vi "StartUp Sequence Open Loop Rev 1.1.vi"() -> ()   [LabVIEW 2017]
panel:
  in  "Shut Off":bool
  out "ECU COM Port Out":refnum<visa-resource-name>
  out "Throttle Position":string
  out "Turbine RPM":string
  out "Turbine Temp":string
  out "Pump Voltage":string
  out "Error Out":errorcluster
  in  "Error In":errorcluster
  in  "ECU COM Port":refnum<visa-resource-name>
  out "Turbine State":string
  in  "Strt Sqnc":bool
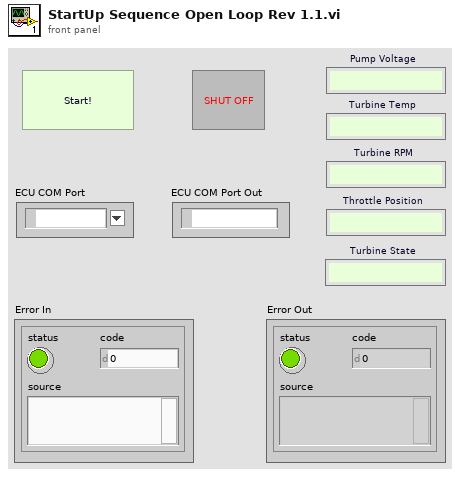
[diagram p1: front panel]
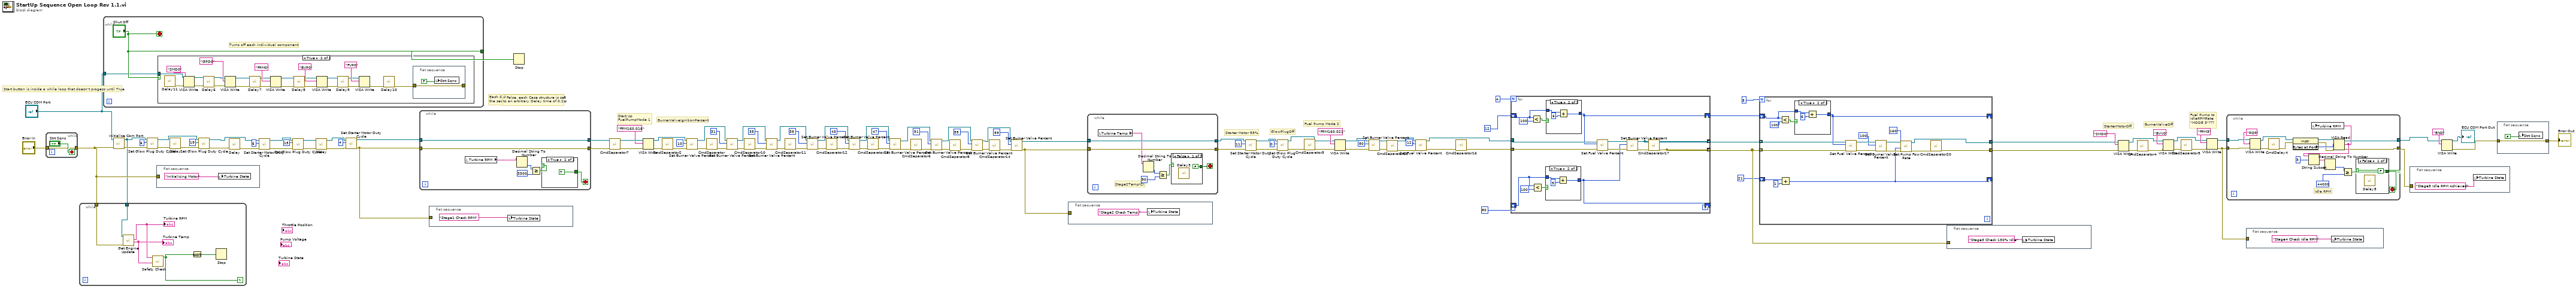
[diagram p0: block diagram]
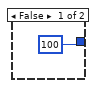
[diagram p2: hidden frame]
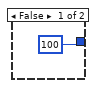
[diagram p3: hidden frame]
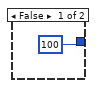
[diagram p4: hidden frame]
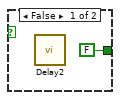
[diagram p6: hidden frame]
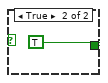
[diagram p7: hidden frame]
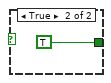
[diagram p8: hidden frame]
diagram:
  # "Start button is inside a while loop that doesn't progess until True"
  # "Fuel Pump Mode 2"
  # "Starter Motor 55%"
  # "Fuel Pump to \nIdleRPMRate\n\"MODE 3\"???"
  # "BurnerValveOff"
  # "StarterMotorOff"
  # "GlowPlugOff"
  # "Start Up\nFuelPumpMode 1"
  # "BurnerValveIgnitionPercent"
  # "If False, each Case structure is set\nto an arbitrary Delay time of 0.2 s"
  # "Each Stage is inside a while loop so that \nthe sequence doesn't progress until True"
  n1 = while {
    tunnel: "Error In" -> [w114]
    tunnel: [w114] -> w2
    stop <- "Strt Sqnc" stop-if-true
  }
  n2 = while {
    tunnel: ["Shut Off"] -> w90
    tunnel: "ECU COM Port" -> [w116]
    stop <- "Shut Off" stop-if-true
    # "Turns off each individual component"
    n3 = case shown="True" "Shut Off" {
      tunnel: w116 -> [_ w120]
      frame False {
      }
      frame True {
        n4 = call "Delay11"() -> ("error out"=w118:errorcluster)  [unwired: 11 in]
        n5 = VISA Write(VISA resource name=w120, write buffer="SMD0", error in (no error)=w118) -> (VISA resource name out=w125:refnum<visa-resource-name>, error out=w138:errorcluster)  [unwired: 1 out]
        n6 = call "Delay6"("error in (no error)"=w138) -> ("error out"=w132:errorcluster)  [unwired: 10 in]
        n7 = VISA Write(VISA resource name=w125, write buffer="GPD0", error in (no error)=w132) -> (VISA resource name out=w123:refnum<visa-resource-name>, error out=w136:errorcluster)  [unwired: 1 out]
        n8 = call "Delay7"("error in (no error)"=w136) -> ("error out"=w131:errorcluster)  [unwired: 10 in]
        n9 = VISA Write(VISA resource name=w123, write buffer="FPM0", error in (no error)=w131) -> (VISA resource name out=w122:refnum<visa-resource-name>, error out=w135:errorcluster)  [unwired: 1 out]
        n10 = call "Delay8"("error in (no error)"=w135) -> ("error out"=w130:errorcluster)  [unwired: 10 in]
        n11 = VISA Write(VISA resource name=w122, write buffer="BVP0", error in (no error)=w130) -> (VISA resource name out=w121:refnum<visa-resource-name>, error out=w134:errorcluster)  [unwired: 1 out]
        n12 = call "Delay9"("error in (no error)"=w134) -> ("error out"=w129:errorcluster)  [unwired: 10 in]
        n13 = VISA Write(VISA resource name=w121, write buffer="FVP0", error in (no error)=w129) -> (error out=w133:errorcluster)  [unwired: 2 out]
        n14 = call "Delay10"("error in (no error)"=w133) -> ("error out"=w119:errorcluster)  [unwired: 10 in]
        n15 = flat-sequence {
          tunnel: w119 -> [w139]
          tunnel: [w139] -> _
          frame #0 {
            n16 = local write "Strt Sqnc"(FALSE ("Strt Sqnc")) -> ()
          }
        }
      }
    }
  }
  n17 = call "Initialize Com Port.vi"("Error In"=w2, "ECU COM Port"="ECU COM Port") -> ("Error Out"=w80:errorcluster, "ECU COM Port Out"=w1:refnum<visa-resource-name>)  [unwired: 8 in]
  n18 = while {
    tunnel: w2 -> [w146]
    tunnel: w1 -> [w145]
    stop <- w142 continue-if-true
    n19 = call "Get Engine Update.vi"("Error In"=w146, "ECU COM Port"=w145) -> ("Temperature"=w143:string, "RPMs"=w144:string)  [unwired: 6 in, 2 out]
    "Turbine RPM" <- w144
    "Turbine Temp" <- w143
    n20 = call "Safety Check.vi"("Temperature"=w143, "RPMs"=w144) -> ("Safe?"=w142:bool)  [unwired: 9 in]
    n21 = Not(x=w142) -> (.not. x?=w141:bool)
    n22 = Stop(stop? (T)=w141) -> ()
  }
  n23 = call "Set Glow Plug Duty Cycle.vi"("Error In"=w80, "Duty Cycle"=6, "ECU COM Port"=w1) -> ("Error Out"=w79:errorcluster, "ECU COM Port Out"=w76:refnum<visa-resource-name>)  [unwired: 7 in]
  n24 = flat-sequence {
    tunnel: w2 -> [_]
    frame #0 {
      n25 = local write "Turbine State"("Initializing Motor") -> ()
    }
  }
  n26 = call "Delay"("error in (no error)"=w79) -> ("error out"=w78:errorcluster)  [unwired: 10 in]
  n27 = call "Set Glow Plug Duty Cycle.vi"("Error In"=w78, "Duty Cycle"=19, "ECU COM Port"=w76) -> ("Error Out"=w77:errorcluster, "ECU COM Port Out"=w72:refnum<visa-resource-name>)  [unwired: 7 in]
  n28 = call "Delay"("error in (no error)"=w77) -> ("error out"=w73:errorcluster)  [unwired: 10 in]
  n29 = call "Set Starter Motor Duty Cycle.vi"("Error In"=w73, "Duty Cycle"=6, "ECU COM Port"=w72) -> ("Error Out"=w71:errorcluster, "ECU COM Port Out"=w69:refnum<visa-resource-name>)  [unwired: 7 in]
  n30 = call "Set Glow Plug Duty Cycle.vi"("Error In"=w71, "Duty Cycle"=15, "ECU COM Port"=w69) -> ("Error Out"=w70:errorcluster, "ECU COM Port Out"=w66:refnum<visa-resource-name>)  [unwired: 7 in]
  n31 = call "Delay"("error in (no error)"=w70) -> ("error out"=w67:errorcluster)  [unwired: 10 in]
  n32 = call "Set Starter Motor Duty Cycle.vi"("Error In"=w67, "Duty Cycle"=4, "ECU COM Port"=w66) -> ("Error Out"=w91:errorcluster, "ECU COM Port Out"=w65:refnum<visa-resource-name>)  [unwired: 7 in]
  n33 = while {
    tunnel: w91 -> [w150]
    tunnel: w65 -> [w149]
    tunnel: [w149] -> w101
    tunnel: [w150] -> w100
    stop <- w153 stop-if-true
    n34 = local read "Turbine RPM"() -> (w148:string)
    n35 = Decimal String To Number(string=w148) -> (number=w152:i32)  [unwired: 2 in, 1 out]
    n36 = Greater Or Equal?(x=w152, y=3300) -> (x >= y?=w154:bool)
    n37 = case shown="True" w154 {
      tunnel: [FALSE TRUE] -> w153
      frame False {
        n38 = call "Delay2"() -> ()  [unwired: 11 in, 1 out]
      }
      frame True {
      }
    }
  }
  n39 = flat-sequence {
    tunnel: w91 -> [_]
    frame #0 {
      n40 = local write "Turbine State"("Stage1 Check RPM") -> ()
    }
  }
  n41 = Stop(stop? (T)=w90) -> ()
  n42 = call "CmdSeparator7"("error in (no error)"=w100) -> ("error out"=w99:errorcluster)  [unwired: 10 in]
  n43 = VISA Write(VISA resource name=w101, write buffer="FPM160,016", error in (no error)=w99) -> (VISA resource name out=w53:refnum<visa-resource-name>, error out=w112:errorcluster)  [unwired: 1 out]
  n44 = call "CmdSeparator2"("error in (no error)"=w112) -> ("error out"=w64:errorcluster)  [unwired: 10 in]
  n45 = call "Set Burner Valve Percent.vi"("Error In"=w64, "Percent"=10, "ECU COM Port"=w53) -> ("Error Out"=w63:errorcluster, "ECU COM Port Out"=w52:refnum<visa-resource-name>)  [unwired: 7 in]
  n46 = call "CmdSeparator"("error in (no error)"=w63) -> ("error out"=w62:errorcluster)  [unwired: 10 in]
  n47 = call "Set Burner Valve Percent.vi"("Error In"=w62, "Percent"=31, "ECU COM Port"=w52) -> ("Error Out"=w61:errorcluster, "ECU COM Port Out"=w51:refnum<visa-resource-name>)  [unwired: 7 in]
  n48 = call "CmdSeparator10"("error in (no error)"=w61) -> ("error out"=w60:errorcluster)  [unwired: 10 in]
  n49 = call "Set Burner Valve Percent.vi"("Error In"=w60, "Percent"=35, "ECU COM Port"=w51) -> ("Error Out"=w59:errorcluster, "ECU COM Port Out"=w50:refnum<visa-resource-name>)  [unwired: 7 in]
  n50 = call "CmdSeparator11"("error in (no error)"=w59) -> ("error out"=w58:errorcluster)  [unwired: 10 in]
  n51 = call "Set Burner Valve Percent.vi"("Error In"=w58, "Percent"=39, "ECU COM Port"=w50) -> ("Error Out"=w57:errorcluster, "ECU COM Port Out"=w49:refnum<visa-resource-name>)  [unwired: 7 in]
  n52 = call "CmdSeparator12"("error in (no error)"=w57) -> ("error out"=w56:errorcluster)  [unwired: 10 in]
  n53 = call "Set Burner Valve Percent.vi"("Error In"=w56, "Percent"=43, "ECU COM Port"=w49) -> ("Error Out"=w55:errorcluster, "ECU COM Port Out"=w48:refnum<visa-resource-name>)  [unwired: 7 in]
  n54 = call "CmdSeparator13"("error in (no error)"=w55) -> ("error out"=w54:errorcluster)  [unwired: 10 in]
  n55 = call "Set Burner Valve Percent.vi"("Error In"=w54, "Percent"=47, "ECU COM Port"=w48) -> ("Error Out"=w24:errorcluster, "ECU COM Port Out"=w23:refnum<visa-resource-name>)  [unwired: 7 in]
  n56 = call "CmdSeparator6"("error in (no error)"=w24) -> ("error out"=w26:errorcluster)  [unwired: 10 in]
  n57 = call "Set Burner Valve Percent.vi"("Error In"=w26, "Percent"=51, "ECU COM Port"=w23) -> ("Error Out"=w19:errorcluster, "ECU COM Port Out"=w20:refnum<visa-resource-name>)  [unwired: 7 in]
  n58 = call "CmdSeparator8"("error in (no error)"=w19) -> ("error out"=w22:errorcluster)  [unwired: 10 in]
  n59 = call "Set Burner Valve Percent.vi"("Error In"=w22, "Percent"=55, "ECU COM Port"=w20) -> ("Error Out"=w15:errorcluster, "ECU COM Port Out"=w16:refnum<visa-resource-name>)  [unwired: 7 in]
  n60 = call "CmdSeparator14"("error in (no error)"=w15) -> ("error out"=w18:errorcluster)  [unwired: 10 in]
  n61 = call "Set Burner Valve Percent.vi"("Error In"=w18, "Percent"=59, "ECU COM Port"=w16) -> ("Error Out"=w89:errorcluster, "ECU COM Port Out"=w14:refnum<visa-resource-name>)  [unwired: 7 in]
  n62 = flat-sequence {
    tunnel: w89 -> [_]
    frame #0 {
      n63 = local write "Turbine State"("Stage2 Check Temp.") -> ()
    }
  }
  n64 = while {
    tunnel: w14 -> [w160]
    tunnel: w89 -> [w161]
    tunnel: [w160] -> w35
    tunnel: [w161] -> w37
    stop <- w164 stop-if-true
    # "Stage2Temp(C)"
    n65 = local read "Turbine Temp"() -> (w159:string)
    n66 = Decimal String To Number(string=w159) -> (number=w162:i32)  [unwired: 2 in, 1 out]
    n67 = Greater Or Equal?(x=w162, y=90) -> (x >= y?=w165:bool)
    n68 = case shown="False" w165 {
      tunnel: [FALSE TRUE] -> w164
      frame False {
        n69 = call "Delay3"() -> ()  [unwired: 11 in, 1 out]
      }
      frame True {
      }
    }
  }
  n70 = call "Set Starter Motor Duty Cycle.vi"("Error In"=w37, "Duty Cycle"=11, "ECU COM Port"=w35) -> ("Error Out"=w36:errorcluster, "ECU COM Port Out"=w34:refnum<visa-resource-name>)  [unwired: 7 in]
  n71 = call "Set Glow Plug Duty Cycle.vi"("Error In"=w36, "Duty Cycle"=0, "ECU COM Port"=w34) -> ("Error Out"=w33:errorcluster, "ECU COM Port Out"=w31:refnum<visa-resource-name>)  [unwired: 7 in]
  n72 = call "CmdSeparator3"("error in (no error)"=w33) -> ("error out"=w32:errorcluster)  [unwired: 10 in]
  n73 = VISA Write(VISA resource name=w31, write buffer="FPM160,021", error in (no error)=w32) -> (VISA resource name out=w28:refnum<visa-resource-name>, error out=w30:errorcluster)  [unwired: 1 out]
  n74 = call "Set Burner Valve Percent.vi"("Error In"=w30, "Percent"=80, "ECU COM Port"=w28) -> ("Error Out"=w13:errorcluster, "ECU COM Port Out"=w27:refnum<visa-resource-name>)  [unwired: 7 in]
  n75 = call "CmdSeparator18"("error in (no error)"=w13) -> ("error out"=w12:errorcluster)  [unwired: 10 in]
  n76 = call "Set Fuel Valve Percent.vi"("Error In"=w12, "Percent"=12, "ECU COM Port"=w27) -> ("Error Out"=w11:errorcluster, "ECU COM Port Out"=w29:refnum<visa-resource-name>)  [unwired: 7 in]
  n77 = call "CmdSeparator16"("error in (no error)"=w11) -> ("error out"=w86:errorcluster)  [unwired: 10 in]
  n78 = for {
    N: 4 -> [_]
    tunnel: [w168] -> _
    tunnel: [w182] -> _
    tunnel: w29 -> [w174]
    tunnel: w86 -> [w175]
    shift-right: [w173] -> w6
    shift-left: 12 -> [w179]
    shift-right: [w170] -> _
    shift-left: 80 -> [w176]
    tunnel: [w182] -> w8 mode=indexing
    tunnel: [w168] -> w7 mode=indexing
    n79 = Less?(x=w179, y=100) -> (x < y?=w180:bool)
    n80 = Less?(x=w176, y=100) -> (x < y?=w177:bool)
    n81 = case shown="True" w177 {
      tunnel: w176 -> [_ w186]
      tunnel: [100 w184] -> w170
      frame False {
      }
      frame True {
        n82 = Add(x=w186, y=5) -> (x+y=w184:i32)
      }
    }
    n83 = case shown="True" w180 {
      tunnel: w179 -> [_ w190]
      tunnel: [100 w188] -> w173
      frame False {
      }
      frame True {
        n84 = Add(x=w190, y=6) -> (x+y=w188:i32)
      }
    }
    n85 = call "Set Fuel Valve Percent.vi"("Error In"=w175, "Percent"=w173, "ECU COM Port"=w174) -> ("Error Out"=w172:errorcluster, "ECU COM Port Out"=w169:refnum<visa-resource-name>)  [unwired: 7 in]
    n86 = call "Set Burner Valve Percent.vi"("Error In"=w172, "Percent"=w170, "ECU COM Port"=w169) -> ("Error Out"=w171:errorcluster, "ECU COM Port Out"=w168:refnum<visa-resource-name>)  [unwired: 7 in]
    n87 = call "CmdSeparator17"("error in (no error)"=w171) -> ("error out"=w182:errorcluster)  [unwired: 10 in]
  }
  n88 = for {
    N: 5 -> [_]
    tunnel: [w197] -> w3
    tunnel: [w208] -> w4
    shift-right: [w204] -> _
    shift-left: w6 -> [w205]
    tunnel: w8 -> [w201] mode=indexing
    tunnel: w7 -> [w200] mode=indexing
    shift-right: [w191] -> _
    shift-left: 21 -> [w192]
    n89 = Less?(x=w205, y=100) -> (x < y?=w206:bool)
    n90 = Add(x=w192, y=1) -> (x+y=w191:i32)
    n91 = case shown="True" w206 {
      tunnel: w205 -> [_ w212]
      tunnel: [100 w210] -> w204
      frame False {
      }
      frame True {
        n92 = Add(x=w212, y=6) -> (x+y=w210:i32)
      }
    }
    n93 = call "Set Fuel Valve Percent.vi"("Error In"=w201, "Percent"=w204, "ECU COM Port"=w200) -> ("Error Out"=w203:errorcluster, "ECU COM Port Out"=w202:refnum<visa-resource-name>)  [unwired: 7 in]
    n94 = call "Set Burner Valve Percent.vi"("Error In"=w203, "Percent"=100 ("y"), "ECU COM Port"=w202) -> ("Error Out"=w195:errorcluster, "ECU COM Port Out"=w198:refnum<visa-resource-name>)  [unwired: 7 in]
    n95 = call "Set Pump Fow Rate.vi"("Error In"=w195, "Pulse Width"=w191, "Voltage"=160 ("y"), "ECU COM Port"=w198) -> ("Error Out"=w196:errorcluster, "ECU COM Port Out"=w197:refnum<visa-resource-name>)  [unwired: 6 in]
    n96 = call "CmdSeparator20"("error in (no error)"=w196) -> ("error out"=w208:errorcluster)  [unwired: 10 in]
  }
  n97 = flat-sequence {
    tunnel: w8 -> [_]
    frame #0 {
      n98 = local write "Turbine State"("Stage3 Check 130% Idle") -> ()
    }
  }
  n99 = VISA Write(VISA resource name=w3, write buffer="SMD0", error in (no error)=w4) -> (VISA resource name out=w107:refnum<visa-resource-name>, error out=w109:errorcluster)  [unwired: 1 out]
  n100 = call "CmdSeparator4"("error in (no error)"=w109) -> ("error out"=w108:errorcluster)  [unwired: 10 in]
  n101 = VISA Write(VISA resource name=w107, write buffer="BVV0", error in (no error)=w108) -> (VISA resource name out=w104:refnum<visa-resource-name>, error out=w103:errorcluster)  [unwired: 1 out]
  n102 = call "CmdSeparator5"("error in (no error)"=w103) -> ("error out"=w105:errorcluster)  [unwired: 10 in]
  n103 = VISA Write(VISA resource name=w104, write buffer="FPM3", error in (no error)=w105) -> (VISA resource name out=w102:refnum<visa-resource-name>, error out=w93:errorcluster)  [unwired: 1 out]
  n104 = while {
    tunnel: w102 -> [w220]
    tunnel: w93 -> [w219]
    tunnel: [w217] -> w92
    tunnel: [w216] -> w95
    stop <- w231 stop-if-true
    # "Idle RPM"
    n105 = VISA Write(VISA resource name=w220, write buffer="RQR", error in (no error)=w219) -> (VISA resource name out=w227:refnum<visa-resource-name>, error out=w229:errorcluster)  [unwired: 1 out]
    n106 = call "CmdDelay4"("error in (no error)"=w229) -> ("error out"=w228:errorcluster)  [unwired: 10 in]
    n107 = property class="Instr"(reference=w227, error in=w228) -> (reference out=w224:refnum<visa-resource-name>, error out=w225:errorcluster, "Bytes at Port"=w226:u32)
    n108 = VISA Read(VISA resource name=w224, byte count=w226, error in (no error)=w225) -> (VISA resource name out=w216:refnum<visa-resource-name>, read buffer=w218:string, error out=w217:errorcluster)  [unwired: 1 out]
    n109 = String Subset(string=w218, offset (0)=3) -> (substring=w222:string)  [unwired: 1 in]
    n110 = local write "Turbine RPM"(w218) -> ()
    n111 = Decimal String To Number(string=w222) -> (number=w221:i32)  [unwired: 2 in, 1 out]
    n112 = Greater Or Equal?(x=w221, y=44000) -> (x >= y?=w215:bool)
    n113 = case shown="False" w215 {
      tunnel: [FALSE TRUE] -> w231
      frame False {
        n114 = call "Delay5"() -> ()  [unwired: 11 in, 1 out]
      }
      frame True {
      }
    }
  }
  n115 = flat-sequence {
    tunnel: w93 -> [_]
    frame #0 {
      n116 = local write "Turbine State"("Stage4 Check Idle RPM") -> ()
    }
  }
  n117 = flat-sequence {
    tunnel: w92 -> [_]
    frame #0 {
      n118 = local write "Turbine State"("Stage5 Idle RPM Achieved") -> ()
    }
  }
  n119 = VISA Write(VISA resource name=w95, write buffer="END") -> (VISA resource name out=→"ECU COM Port Out":refnum<visa-resource-name>, error out=w88:errorcluster)  [unwired: 1 in, 1 out]
  n120 = flat-sequence {
    tunnel: w88 -> [w236]
    tunnel: [w236] -> w87
    frame #0 {
      n121 = local write "Strt Sqnc"(FALSE ("Strt Sqnc")) -> ()
    }
  }
  "Error Out" <- w87
